vi "Get Temperature.vi"(8 "error in (no error)":errorcluster, 11 "UV-VIS in":refnum<class "CCD_camera.lvclass">) -> (0 "error out":errorcluster, 2 "Temperature":i32, 3 "UV-VIS out":refnum<class "CCD_camera.lvclass">)   [LabVIEW 2018, in "CCD_camera.lvclass"]
uses:
  CCD_camera.lvclass
  C:/Users/Sergey Denisov/Documents/REPS/TRANCON/Classes/Detector/Detector.lvclass
  dependecies/Error Code Enum typedef.ctl
  Detector.lvclass/Detector.ctl
  Detector.lvclass
panel:
  out "DLL error code":u32
  out "status":T1
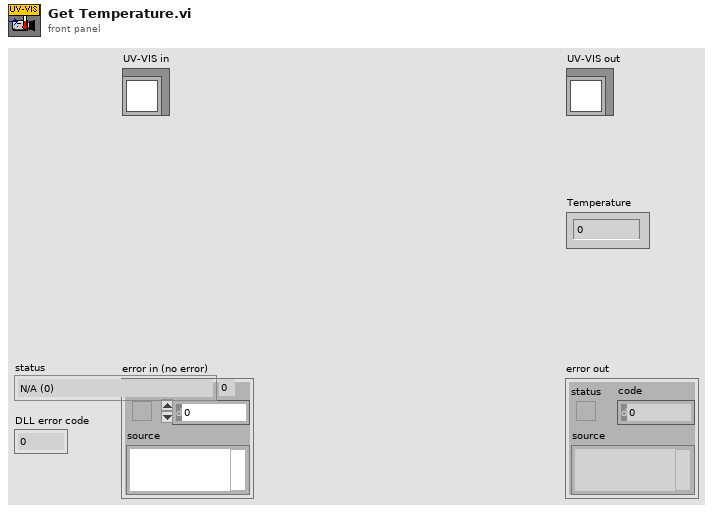
[diagram p1: front panel]
types:
  T1 = typedef "Error Code Enum typedef.ctl" = enum32{"N/A (0)", "DRV_ERROR_CODES", "DRV_SUCCESS", "DRV_VXDNOTINSTALLED", "DRV_ERROR_SCAN", "DRV_ERROR_CHECK_SUM", "DRV_ERROR_FILELOAD", "DRV_UNKNOWN_FUNC", "DRV_ERROR_VXD_INIT", "DRV_ERROR_ADDRESS", "DRV_ERROR_PAGELOCK", "DRV_ERROR_PAGEUNLOCK", "DRV_ERROR_BOARDTEST", "DRV_ERROR_ACK", "DRV_ERROR_UP_FIFO", "DRV_ERROR_PATTERN", "N/A (16)", "DRV_ACQUISITION_ERRORS", "DRV_ACQ_BUFFER", "DRV_ACQ_DOWNFIFO_FULL", "DRV_PROC_UNKONWN_INSTRUCTION", "DRV_ILLEGAL_OP_CODE", "DRV_KINETIC_TIME_NOT_MET", "DRV_ACCUM_TIME_NOT_MET", "DRV_NO_NEW_DATA", "N/A (25)", "DRV_SPOOLERROR", "N/A (27)", "N/A (28)", "N/A (29)", "N/A (30)", "N/A (31)", "N/A (32)", "DRV_TEMPERATURE_CODES", "DRV_TEMPERATURE_OFF", "DRV_TEMPERATURE_NOT_STABILIZED", "DRV_TEMPERATURE_STABILIZED", "DRV_TEMPERATURE_NOT_REACHED", "DRV_TEMPERATURE_OUT_RANGE", "DRV_TEMPERATURE_NOT_SUPPORTED", "DRV_TEMPERATURE_DRIFT", "N/A (41)", "N/A (42)", "N/A (43)", "N/A (44)", "N/A (45)", "N/A (46)", "N/A (47)", "N/A (48)", "DRV_GENERAL_ERRORS", "DRV_INVALID_AUX", "DRV_COF_NOTLOADED", "DRV_FPGAPROG", "DRV_FLEXERROR", "DRV_GPIBERROR", "N/A (55)", "N/A (56)", "N/A (57)", "N/A (58)", "N/A (59)", "N/A (60)", "N/A (61)", "N/A (62)", "N/A (63)", "DRV_DATATYPE", "DRV_DRIVER_ERRORS", "DRV_P1INVALID", "DRV_P2INVALID", "DRV_P3INVALID", "DRV_P4INVALID", "DRV_INIERROR", "DRV_COFERROR", "DRV_ACQUIRING", "DRV_IDLE", "DRV_TEMPCYCLE", "DRV_NOT_INITIALIZED", "DRV_P5INVALID", "DRV_P6INVALID", "DRV_INVALID_MODE", "DRV_INVALID_FILTER", "DRV_I2CERRORS", "DRV_I2CDEVNOTFOUND", "DRV_I2CTIMEOUT", "DRV_P7INVALID", "N/A (84)", "N/A (85)", "N/A (86)", "N/A (87)", "N/A (88)", "N/A (89)", "DRV_IOCERROR", "DRV_VRMVERSIONERROR"}
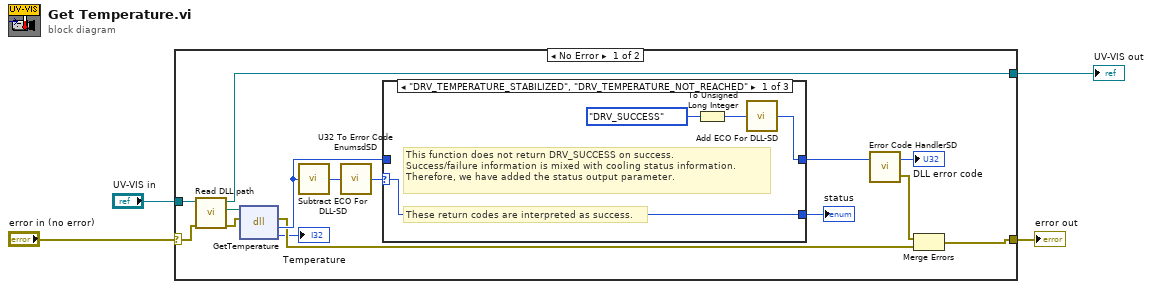
[diagram p0: block diagram]
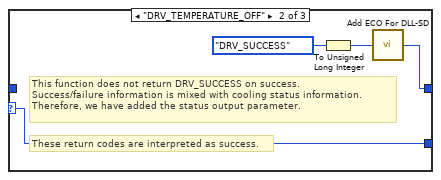
[diagram p2: hidden frame]
diagram:
  n1 = case shown="No Error" "error in (no error)" {
    selector: "error in (no error)" -> [w13 w31]
    tunnel: [w8 w31] -> w1
    tunnel: [w5 w30] -> w2
    tunnel: "UV-VIS in" -> [w7 w30]
    frame No Error {
      n2 = call "Read DLL path.vi"("error in (no error)"=w13, "Detector in"=w7) -> ("error out"=w12:errorcluster, "DLL path"=w11:path, "Detector out"=w5:refnum<class "CCD_camera.lvclass">)  [unwired: 7 in]
      n3 = dll-call lib="G:/SD/TRANCON/DLL/Atmcd32d.dll" fn="GetTemperature"(path in=w11, error in=w12) -> (error out=w9:errorcluster, "type de retour"=w14:u32, "temperature"=→"Temperature":i32)  [unwired: 2 in, 1 out]
      n4 = call "Subtract ECO For DLL-SD.vi"("x"=w14) -> ("x - ECO4DLL"=w18:u32)
      n5 = call "U32 To Error Code EnumsdSD.vi"("U32"=w18) -> ("error code enum"=w17:T1)
      n6 = case shown="\"DRV_TEMPERATURE_STABILIZED\", \"DRV_TEMPERATURE_NOT_REACHED\"" w17 {
        selector: w17 -> [w23 w27 w28]
        tunnel: [w23 w27 w28] -> w16
        tunnel: w14 -> [_ _ w29]
        tunnel: [w20 w24 w29] -> w15
        frame "DRV_TEMPERATURE_STABILIZED", "DRV_TEMPERATURE_NOT_REACHED" {
          # "These return codes are interpreted as success."
          # "This function does not return DRV_SUCCESS on success.\nSuccess/failure information is mixed with cooling status information.\nTherefore, we have added the status output parameter."
          n7 = To Unsigned Long Integer(number=Error_Code_Enum_typedef."DRV_SUCCESS" ("error code enum")) -> (unsigned 32bit integer=w21:u32)
          n8 = call "Add ECO For DLL-SD.vi"("x"=w21) -> ("x + ECO4DLL"=w20:u32)
        }
        frame "DRV_TEMPERATURE_OFF" {
          # "These return codes are interpreted as success."
          # "This function does not return DRV_SUCCESS on success.\nSuccess/failure information is mixed with cooling status information.\nTherefore, we have added the status output parameter."
          n9 = To Unsigned Long Integer(number=Error_Code_Enum_typedef."DRV_SUCCESS" ("error code enum")) -> (unsigned 32bit integer=w25:u32)
          n10 = call "Add ECO For DLL-SD.vi"("x"=w25) -> ("x + ECO4DLL"=w24:u32)
        }
        frame Default {
          # "These return codes are interpreted as errors."
        }
      }
      "status" <- w16
      n11 = call "Error Code HandlerSD.vi"("DLL error code"=w15) -> ("error out"=w10:errorcluster, "dup DLL error code"=→"DLL error code":u32)  [unwired: 1 in]
      n12 = Merge Errors(w10, w9) -> (w8:errorcluster)
    }
    frame Error {
    }
  }
  "error out" <- w1
  "UV-VIS out" <- w2
